vi "1_SimpleDemo_MHHisto.vi"() -> ()   [LabVIEW 2010]
uses:
  _lib/PQ/MultiHarp/mhlib_x86_x64_UIThread.llb/MH_DllPath_global.vi
  _lib/PQ/MultiHarp/MH_RefSource.ctl
  _lib/PQ/MultiHarp/MH_LibVersion_global.vi
  _lib/PQ/MultiHarp/MH_MeasMode.ctl
panel:
  in  "Binning":i32(ring) caption="Resolution [ps]" items=["80", "160", "320", "640", "1280", "2560", "5120", "10240", "20480", "40960", "81920", "163840", "327680", "655360", "1310720", "2621440", "5242880", "10485760", "20971520", "41943040", "83886080", "167772160", "335544320"]
  in  "HistoLength":i32(ring)=6 caption="Histo Length" items=["1024", "2048", "4096", "8192", "16384", "32768", "65536"]
  in  "Acqu.Time":i32=10000 caption="Acqu.Time [ms]" min=1 max=360000 step=1
  in  "GlobalOffset":i32 caption="GlobalOffset [ns]" min=0 max=100000000 step=1
  in  "OverflowLevel":u32=65535 min=1 step=1
  in  "StopOnOverflow":bool=TRUE
  in  "Trg.Edge":i32(ring) items=["falling", "rising"]
  in  "Trg.Level":i32=-50 caption="Trg.Level [mV]" min=-1200 max=1200 step=1
  in  "Offset":i32 caption="Offset [ps]" min=-99999 max=99999 step=1
  in  "Enable":bool=TRUE
  in  "SyncTrg.Edge":i32(ring) items=["falling", "rising"]
  in  "SyncTrg.Level":i32=-50 caption="SyncTrg.Level [mV]" min=-1200 max=1200 step=1
  in  "SyncOffset":i32 caption="SyncOffset [ps]" min=-99999 max=99999 step=1
  in  "SyncDivider":i32(ring)=8 items=["1"=1, "2"=2, "4"=4, "8"=8, "16"=16]
  out "HistoGraph":T1(graph)={0.0, "Resolution"=0.08, "Histogram"=[]}
  out "CountRates":i32[](array[numeric]) caption="Count Rates [cps]"
  out "SyncRate":i32 caption="Sync Rate [cps]"
  in  "stop":bool
  out "error out":errorcluster
  # "Acquisition"
  # "All Channels"
  # "Sync"
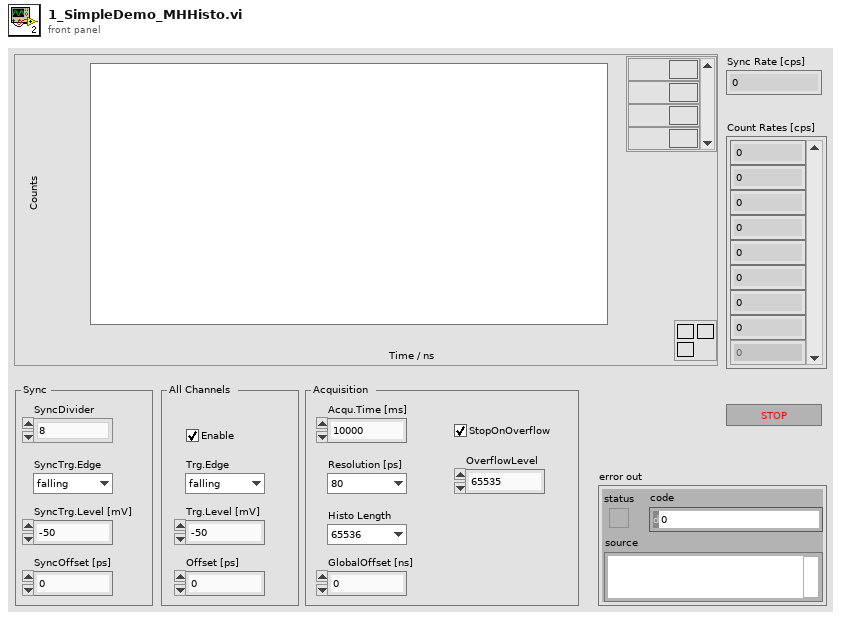
[diagram p1: front panel]
types:
  T1 = cluster{dbl, "Resolution":dbl, "Histogram":u32[][]}
  T2 = typedef "MH_MeasMode.ctl" = i32
  T3 = typedef "MH_RefSource.ctl" = enum16{"INTERNAL", "EXTERNAL_10MHZ", "WR_MASTER_GENERIC", "WR_SLAVE_GENERIC", "WR_GRANDM_GENERIC", "EXTN_GPS_PPS", "EXTN_GPS_PPS_UART", "WR_MASTER_MHARP", "WR_SLAVE_MHARP", "WR_GRANDM_MHARP"}
  T4 = typedef "MH_InitInfo.ctl" = cluster{"Library Version":string, "Serial No.":string, "Model":string, "Partnum":string, "Version":string, "features":i32, "nchannels":i32, "Base Resolution":dbl, "Bin Steps":i32}
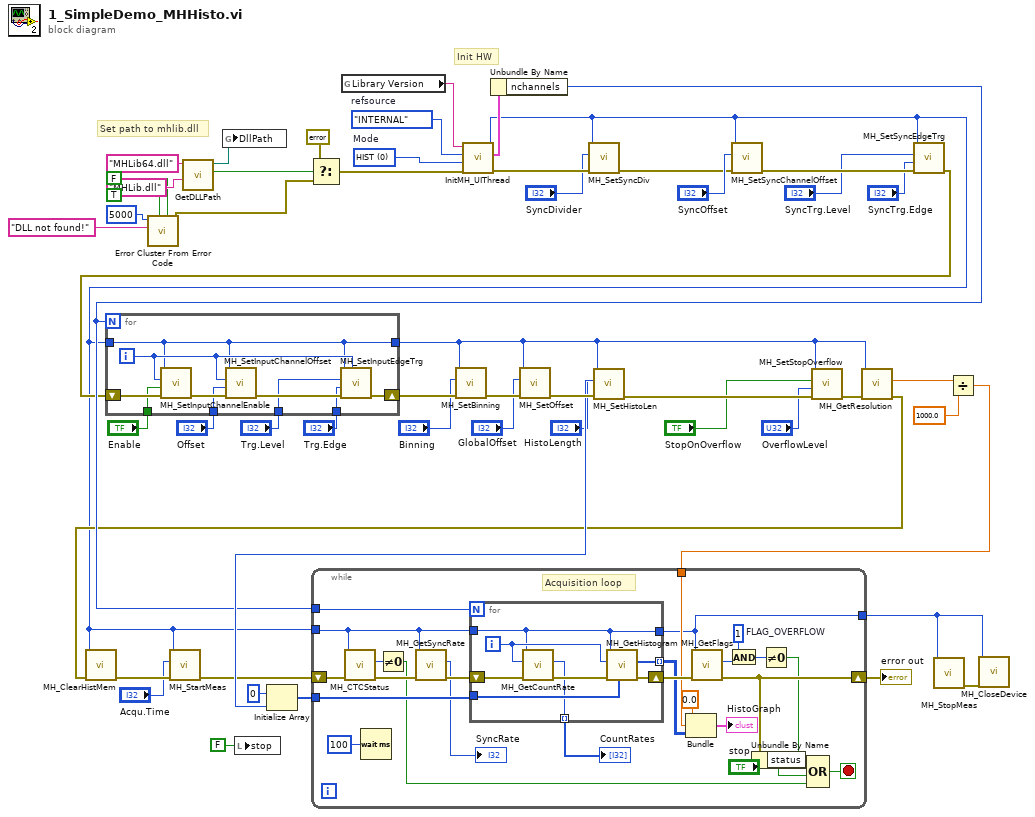
[diagram p0: block diagram]
diagram:
  w5 = T2 0 items=["HIST"=0, "T2"=2, "T3"=3]  # Mode
  w54 = MH_RefSource."INTERNAL"  # refsource
  # "Init HW"
  # "Set path to mhlib.dll"
  n1 = call <vilib>:"Error Cluster From Error Code.vi"("is warning? (False)"=FALSE, "show call chain? (False)"=TRUE, "error message (\"\")"="DLL not found!" ("error message (\"\")"), "error code (0)"=5000) -> ("error out"=w53:errorcluster)  [unwired: 5 in]
  n2 = call "GetDLLPath.vi"("DllName_32bit"="MHLib.dll" ("name or relative path"), "DllName_64bit"="MHLib64.dll" ("name or relative path")) -> ("file exists?"=w51:bool, "DLLPath"=w50:path)  [unwired: 8 in]
  n3 = global write "MH_DllPath_global.vi" "DllPath"(w50) -> ()
  n4 = local write "stop"(FALSE ("stop")) -> ()
  n5 = Select(t=errorcluster {"status"=FALSE, "code"=0, "source"=""} ("error IO"), s=w51, f=w53) -> (s? t:f=w47:errorcluster)
  n6 = global read "MH_LibVersion_global.vi" "Library Version"() -> (w8:string)
  n7 = call "InitMH_UIThread.vi"("error in (no error)"=w47, "Mode"=w5, "refsource"=w54, "Library Version"=w8) -> ("error out"=w41:errorcluster, "Init Info"=w43:T4, "DevIdx"=w14:i32)  [unwired: 5 in]
  n8 = Unbundle By Name(w43) -> ("nchannels"=w23:i32)
  n9 = call "MH_SetSyncDiv.vi"("error in (no error)"=w41, "SyncDivider"="SyncDivider", "devidx"=w14) -> ("error out"=w40:errorcluster)  [unwired: 7 in, 1 out]
  n10 = call "MH_SetSyncChannelOffset.vi"("error in (no error)"=w40, "Offset"="SyncOffset", "devidx"=w14) -> ("error out"=w45:errorcluster)  [unwired: 7 in, 1 out]
  n11 = call "MH_SetSyncEdgeTrg.vi"("error in (no error)"=w45, "edge"="SyncTrg.Edge", "level"="SyncTrg.Level", "devidx"=w14) -> ("error out"=w22:errorcluster)  [unwired: 6 in, 1 out]
  n12 = for {
    N: w23 -> [_]
    shift-right: [w61] -> w42
    shift-left: w22 -> [w64]
    tunnel: w14 -> [w59]
    tunnel: [w59] -> w17
    tunnel: "Enable" -> [w58]
    tunnel: "Offset" -> [w57]
    tunnel: "Trg.Edge" -> [w56]
    tunnel: "Trg.Level" -> [w55]
    i -> [w60]
    n13 = call "MH_SetInputChannelEnable.vi"("error in (no error)"=w64, "enable"=w58, "channel"=w60, "devidx"=w59) -> ("error out"=w63:errorcluster)  [unwired: 6 in, 1 out]
    n14 = call "MH_SetInputChannelOffset.vi"("error in (no error)"=w63, "Offset"=w57, "channel"=w60, "devidx"=w59) -> ("error out"=w62:errorcluster)  [unwired: 6 in, 1 out]
    n15 = call "MH_SetInputEdgeTrg.vi"("channel"=w60, "error in (no error)"=w62, "edge"=w56, "level"=w55, "devidx"=w59) -> ("error out"=w61:errorcluster)  [unwired: 5 in, 1 out]
  }
  n16 = call "MH_SetBinning.vi"("error in (no error)"=w42, "Binning"="Binning", "devidx"=w17) -> ("error out"=w38:errorcluster)  [unwired: 7 in, 1 out]
  n17 = call "MH_SetOffset.vi"("error in (no error)"=w38, "Offset"="GlobalOffset", "devidx"=w17) -> ("error out"=w36:errorcluster)  [unwired: 7 in, 1 out]
  n18 = call "MH_SetHistoLen.vi"("error in (no error)"=w36, "lencode"="HistoLength", "devidx"=w17) -> ("error out"=w35:errorcluster, "actuallen"=w28:i32)  [unwired: 6 in, 1 out]
  n19 = Initialize Array(u32 0, w28) -> (w27:u32[])
  n20 = call "MH_SetStopOverflow.vi"("error in (no error)"=w35, "stopcount"="OverflowLevel", "StopOnOverflow"="StopOnOverflow", "devidx"=w17) -> ("error out"=w18:errorcluster)  [unwired: 6 in, 1 out]
  n21 = call "MH_GetResolution.vi"("error in (no error)"=w18, "devidx"=w17) -> ("error out"=w15:errorcluster, "resolution"=w16:dbl)  [unwired: 7 in, 1 out]
  n22 = call "MH_ClearHistMem.vi"("error in (no error)"=w15, "devidx"=w14) -> ("error out"=w32:errorcluster)  [unwired: 8 in, 1 out]
  n23 = call "MH_StartMeas.vi"("error in (no error)"=w32, "tacq"="Acqu.Time", "devidx"=w14) -> ("error out"=w13:errorcluster)  [unwired: 7 in, 1 out]
  n24 = Divide(x=w16, y=1000.0) -> (x/y=w24:dbl)
  n25 = while {
    shift-right: [w77] -> w30
    shift-left: w13 -> [w88]
    tunnel: w14 -> [w84]
    tunnel: w23 -> [w87]
    tunnel: w27 -> [w79]
    tunnel: w24 -> [w71]
    tunnel: [w66] -> w7
    stop <- w78 stop-if-true
    w82 = 1  # FLAG_OVERFLOW
    # "Acquisition loop"
    n26 = call "MH_CTCStatus.vi"("error in (no error)"=w88, "devidx"=w84) -> ("error out"=w86:errorcluster, "ctcstatus"=w89:i32)  [unwired: 7 in, 1 out]
    n27 = Wait (ms)(milliseconds to wait=u32 100) -> ()  [unwired: 1 out]
    n28 = Not Equal To 0?(x=w89) -> (x != 0?=w68:bool)
    n29 = call "MH_GetSyncRate.vi"("error in (no error)"=w86, "devidx"=w84) -> ("error out"=w85:errorcluster, "syncrate"=→"SyncRate":i32)  [unwired: 7 in, 1 out]
    n30 = for {
      N: w87 -> [_]
      shift-right: [w97] -> w83
      shift-left: w85 -> [w96]
      tunnel: w84 -> [w93]
      tunnel: [w93] -> w66
      tunnel: w79 -> [w92]
      tunnel: [w91] -> w74 mode=indexing
      tunnel: [w90] -> w73 mode=indexing
      i -> [w94]
      n31 = call "MH_GetCountRate.vi"("error in (no error)"=w96, "Channel"=w94, "devidx"=w93) -> ("error out"=w95:errorcluster, "rate"=w91:i32)  [unwired: 6 in, 1 out]
      n32 = call "MH_GetHistogram.vi"("Chcount"=w92, "error in (no error)"=w95, "channel"=w94, "devidx"=w93) -> ("error out"=w97:errorcluster, "Histogram"=w90:u32[])  [unwired: 5 in, 1 out]
    }
    "CountRates" <- w74
    n33 = Bundle(0.0, w71, "Histogram"=w73) -> (→"HistoGraph":cluster{dbl, dbl, "Histogram":u32[][]})  [unwired: 1 in]
    n34 = call "MH_GetFlags.vi"("error in (no error)"=w83, "devidx"=w66) -> ("error out"=w77:errorcluster, "flags"=w80:i32)  [unwired: 7 in, 1 out]
    n35 = And(x=w82, y=w80) -> (x .and. y?=w81:i32)
    n36 = Unbundle By Name(w77) -> ("status"=w65:bool)
    n37 = Not Equal To 0?(x=w81) -> (x != 0?=w76:bool)
    n38 = Compound Arithmetic op=OR(w65, w76, "stop", w68) -> (w78:bool)
  }
  "error out" <- w30
  n39 = call "MH_StopMeas.vi"("devidx"=w7) -> ("error out"=w6:errorcluster)  [unwired: 9 in, 1 out]
  n40 = call "MH_CloseDevice.vi"("error in (no error)"=w6, "devidx"=w7) -> ()  [unwired: 8 in, 2 out]
